vi "Main_14a.vi"() -> ()   [LabVIEW 2023]
uses:
  ENUM_Type.ctl
panel:
  out "End":T1[][](array[typedef])
  out "Start":T1[][](array[typedef])
  out "Answer":i32
  in  "Puzzle":string="O.OO.#...#.O#...#...O..O.#O..O.##.....###O.O##O.O....OO.....##..##.#..O#.........O#..#..O...#O.....O\n.....###.O....#.#O.....##..O##O.......##......O..#..##.#.O#...O...O.O....#.###O.OO#.#O.#.#..O..OOO..\nOO......#.#..##O........O.###..#.#........O#..O....O#.#.##.OO.....O#.........###O......#..#.O..#....\n..#O...O....#.#.#O#....#.O#....OO.OO.O#...O##.O........O.#O.OO.O.....O.#.O.#....O.....O..OO.OO...O.#\n..#O...#.....O#O...###O......O#.##O..O#.O.O.#..#O#.O....O..O#...OO...O..#.O.......O.##OO.#...#...##.\n.#......O.OO#....O#O#OO.O..O......OOO..O....O....#OO....O...#.O.O.O..O...OOOO...#......O..#O..#O....\n..O.#.O.#..OO...........#..#......#.#...#...O...#...#...O##..O..#..O.#...O..#.O...#....#..OO..O..#.#\n.##..O..##O......#...##....#..#..O....#..##.#.O#....O#..#...O.O....O.O.........OO.#.OO......O.......\n..##O.O...O.O..O##OO..#.O..O.#...O..#..#.O...O....##...#O...O......#.....O##O#..O.#..#..O...#...#.O.\nO..##...##...#.#.OO#...OO#O..O...O.#O..#.O......O##......#O..O..OOOOOO..O.##.O...#O.....O##......OO.\n.........O..O#.....#...#......OO###OO.O.O#...#.O....O..##..O#.....O.#.##O.#......#.O.....OO#.#..##O.\nOO#O...#...OO.O####.OO.#.#.......O......O#..O#..#...#O....#.....OO#O......#O#...O#.OO......O....O#..\n.O.........#.#O#....#OO..#.........OO....O...#.O.O.O.OOO.O..O.....O.#....OOOO....OO.......#.#.O.##..\n....#.....#.O.#O...O#OO#...##.#.#..O.O.O....#O.#.#.O...#O#O.O#O...O..#OO..O###.OO..#.....OOO.#......\n#OOO..OO.O.O..O..O....#....O..O.#...O...O...##.O##..O...OOOOO#.........OOO##..#...OO#O#O.....O...##.\n.......O#..#OO.O.O..OO.O#..O.......##....OO#.O..O..O#...#..#...O.##.....#..........#.....#.O...#...O\n......O.#.O...O.......O#..O..OOO#...#........###.O..#....O.O#.OO.O..#.O#O.O.O.......O.##.OO......O.#\nO....O..........#....##.###..#...O#.O..O.##.O....O..O..O..##.O.O#OO...O.#.O##..#.#.......#.O..O..O.O\n..O#..O.#.##..O#..O#..O..O..O....OO...O##..#...O.OO..#.#.#.###O.O...#O.##..#.....#..#O.O.O...#O.O#..\n..O.##........OO.....OO.O..#.....OO.O..#...#..OOO..#....#....#.OO.#.#........OO...O.#O....##O..OOOO#\n.........#.#.OO.#O...#...O#........O..#.#........O......O#.OO..#..#....O##OO.......O..O.O.O.........\n#..O..#..OO.O.O....O..O.O.#.O.O#O...O.OO..#......OO.#..O....#.....#OOO#.OO#.OO........###....O.....O\n..O..O.O.O.....O..#.O..##.O..##..O###........O.O..#...O....OOO#.OO.#O...O..##....#.#O...#..O...O...#\nO#...O..O.#.#......O..O.#OO.....O..#.......O.##O........#O.OO..#..O.##..O.#...O...#O.....#.#..OO##..\nO.OO..O....O.#..O##O.#.O.O#O..##...O..##...#.O#.....O##.#O..O.O.....O....##..O.###......#........O..\n.....##.#.......O.OO....#..##............##..O..#.......O..O..#.O...O#..O.O.##..O..OO.O.....O...O...\n##.O.#....O..OO..OOO.OO.##..OO.OO.#...O#.....#...##...O#....OO..O.O...O...O.#....OO...#..#O#.##..#..\n........OOO....O...#.O...O..#......O....#O#.#O...O#.O........O.O...OO#....O..#.#.#O.O...OO....O.#O..\nOO...O...O..#.OO..O#.OO###..O.......#..O..O.####O....O.O.O#O.#..O..##OO..O..#....#..O#O....#..O...O.\n..O....#.O.O....O...#.........#..O#.#..OO....#...##.OO..OO.O...OOO..O..O#.###.......O#...#....OO...#\n.O...OO.O.O...#.......#.O.O.....O...OOOO.#O.O..O..OOO.OO...............#O...##O..OOO##....#O.O#.##..\nO....O...O.#...........#..#.#OO###O.O...#.O#..O.....O...O....O...#...O.OOO.OO#..OO...#..OOOO...#..#.\n....O...OO.#.O...O..#....O.O.#O..O....O..O..##O.#O....O..O.....O.......OO.......#OO#.##.O.#.O..#.##O\n#OO#.#....###O#..OO..#..O.......O.O...OO#.#O.....O.O##.O...#.##O#...O#......#..#..O#O.O.....OO.O#.O.\n...O#....O...O......#..O#O..OO.O#.OO.#.......#...O..O.....O.#O..O..O.....#OO#.O..#....#O.#O..#......\n..O.....O.......#O....O#...##.....#..O.#....#.#.#O#.#....O....#..O.O......OO....O.#OO#OO.....O......\n.#..O..#..O##...#O.#.##O#.#.#O....O#..###.OO..##..#..........O#O.#..#....O...##.......O.O.O##O#..#O.\n.#.....O..O.#..#..O....O...#.....#O.O.....OO.#..#......##........O.#.#......#...OO#....O#O.....#..O#\n#.....O.....O...O..##O.OO#OO......O#..O......O...O...#.....OO..#...O..#.....##.#.O...#..#O......OO.O\n.#..#.#.#...O#.......#.O....O..#.#.#.....O...................#.O...OOO#.....O.O.....O..O.#.....#.O.O\nO....O.....O.....O#O...O.O.O#O.#O..OO#OO..#OO.OO##.....##O#.O.O..#.....O..OO.##.#.......#...O..OO.O.\n.O#..O..#....##......O....#.#.#......#........##...#....#.......#.....O......##.#.....O.O....OO#.O..\n....OO.OO#...O..#O#O.#.O.#..OO...OOO...#O.#..#..#.#O...#O.#.O..##..O.##..O#.#.....#..O...#.O...O#.O#\n....O#....O.O#OOO...#.#.........O.O....#..O...#...#.....O.O.O.O....#.OO.##O.....#.#.#.#O..O#.O.#.OOO\nO#OO..O.#.......###..OO..O........O.##O.#O##..O...O.#OO.....#...O......O.OO...O..OO....O..O..#.#...O\n.#.O.O.O.#......O......##O...OO.....O....O#.....O#....#.......#O..#...##..O..#O.O.O..O....O.........\n...#.........OO..O.O#..O.#....#...OO##...O..OO.......#.#OO..#...#..##.#...OO#...#O.#...O.....O...#..\n#.....#O......O....O#.....#.#O.OO..........O.O...#....#.###O.O..O...#...#..#....O..O..O#.O.........#\nO.O.O...O...#.....#.#....O.O.O.....OO....#..OOO......O.O.......O#O...#.#O##O.####.........O#O.......\nO.O...........O#...OO..#O.O.O......O.......##.O...O..##...O.#OO...#OO...#...#O#.##O.#......O.##....O\nO..#...........O..O......OOO....#....OO.O...#O..O.O#......#...........#O...#O..O....#.#.#..#...#O...\n..O.....#...#...O.#.O..##.........O#..##.....#O.........................##...#.#..#.OO#O...#OOO#O.##\nOO..O.O.....O#.O....O##...O.O#.OO.#..O.....O...##.O#..O......OO..#..O.....##.....OO#OO...#O......O.O\n.OO...#....#O..#.....OO..O.O.......O#...O#..O#..#.O....#.O.#.O...O.#.O.#...#..OO.......O#....OO..O..\nO.OO..#.OOO.#.O#...#.#..O..O#.#.#.#.....#.O#..O....O..OO...O..#..#....OO#O.#......O#..##...O...O.#O.\n....#....#...OO#...O.O#OO.#.#OOO..O...OO.O..#.O#..#..O.O..#.#........OO#O.#.#.#.....OO......##.#.O..\n.#.O.OOO#OOO...##O#.#...#...##O.#...O.......###O#.##..O#..#.##...O..O.O.........O..#..O##......#.##.\nO...#..#....#O..##..O.O##..O.O###O.......O...#.O#.O#..O...#.#.O..#.....#.....O..O..OOO.OOO..O..OOO..\n...O#.O....O.O.#.O..#.O..####...OO......#OO....O#....O..O...O...OO..OO.OOO#....#..#.O.O..#..#.....O.\nO.O##O.O.O.#.O.#........#O......#O.##...##OO.......O#..#..#.O....OO........#.#O..#O.........OO.O#..O\n.......#.....O...O.O.#O##.O.OO#.....O.O#O....O.#.##.#.......##.O.O.###O...O.O#O##...#...#...O..#....\n.O#...#O...#....O##.O..........O.O.#..O.O..OOOOO.......OO.O#...O...O...#O###OOO.#OOO..............O#\nO.#.#.......OO..OO.#.O#.....#.O#O...#......O....O...O.O.....OO.#O.......#..O...O.....##OO#.....OO#.#\n...O#...#.....#..#O.#..O..O.#O#O.#...OO#O.O....O.#...#O#O....#......O..#O...#....O..O.O........#..#.\n.O.......#..O#...O....................#.##O......#.#......####..OO#...OO.##..#........#.OO..#OOO.###\n......O...O..O##.......O...O##O.O....#..#.##...#OO..##..........#..............##O.......O...#O###O.\n.........#..OO.#.......OO...O....#O.#.......O..##...###..O...#OO.O.O...#...#OO....##O.....#O.O..#...\n..#....O..O......#.#....OO#....#...O.#.OO.O#.....O#.#......O.#O.........O....O....#..O.........O....\n.OO.......#.....O.O..O#....O.#.....O..O#O...O#.....OOO....##..O.O..O#.OO...#....#...O..#..##..#..#.O\nO..#..OO##.#..OOO..#...#.OOO..O..##..O..##O.......O.O..O...#.O...#..###.#.#.#...#O..O......#.O#....#\n...O..#O..O..OO.#....#...##...O...#.......OOOO#...O.###.O.......#O.O#.##.##O..#...O...O.O..#....OO..\nOO.........OO...O.O............O....O.O...O.O.O.......O.OOO.O#....#O.O..#.....O#...#...#....#......O\n#.OO#........OO..#OO.....O.#...#..#O.O...O.....#..O.......O...O..O...O.O.O....##...O....O.OO.....#.O\n..O....#..O....O#.....#..#O......O......#...#O.......O.O...##O.#...O#..O#.#O###...#.OOO.#O...O#....O\n.#.#..OO.#..O###....O.#......O..OO...O.O..O.#.O....O.#..O.....O#....O....#.......O.O...O......OOO.#.\n...OO#.OO#O....O....O.O.#.O.#O..#.O#...###...#......#...OO##.#.#..O#...#....#.#.#.OO....O...OOOO...O\n..O.#..O...O...O#O......##.....O...O..O....#....O..#OO.#.O......#O.OOO.O.O..#........##...#O.#O...O.\n..O.OO.....O...#..O..#...O...O..#O..O#..##.....#....#.#O.#.......#O##....O.OOOOOOOO#.O...O.O#..#O##.\nO.OO.####..OO...OO.O........OO#.O.O...#....#..OO......O.O...O..#.##....O....O......#O........#O.O#..\n.#O.#...#.#...OO#.O.#O.....O##.O.OO.O..#..#O.....O...#.O.O#.....###.....#O.O.......O.#O.O#..#.O..#..\n.O......O........O...#O....##.....#O..OO.O..#.....O.#..O...#O#.#..##.#O..........O.O.O..#....#..#..#\n.OOO..O...#O.O#..#....O......O.O...O#O.....#..OO......OO.#O..O..O###......O.#.#.#.O....#...O........\n.##.....#OO#.##.....#....O..O.....OO..OO##...O...O#.##.OO#....#.......#...O.O.#.O........OO...OO....\n......OO#.....OO#OO......#.O....##..O.O#...O....#..O.O.#O.#...#.O..#.O.O#O....O.O..O.O.O.#OO.##.OO.#\n.O..OO##....O###......####.OO...O#..#..##.##.O..#..##OOO...#..#O##.#..#........#...#....O.......#.OO\n..O..O.O..#....#.#O.#.#OOO....O.##.....OO....#..O...#...#O.........O....O..#..........#.O..O.OO.O##O\nOO.......#...O#.#.......O...O.OO#.O.O.....O.....#...##..#....#.......O#.#O..O.O.......##...OO..#O...\n#O#....#.#.O..#...OO...##.#.#.O#O#...#........O..OO..#..O#..O..O.O.#O...#.....#O.#O.O#..OOO#.O.O..#.\n.#O...OO.##.#.....O...O#O................O.O..O#...#..O.#OO..O....OO...O.#...O#.#.O...O#....OO#.#...\nO#...###.OO.O...O.O#O#..O.O...O.#.....O......O...#...O.O....#...O...O#.#...##....O...........#O...#.\n.....#OO.#.OO...##.O....#OO#.....O..##...OO#.......O...##..#....#..#..##.#O.O##..O.#.O.#.O#OO.O.#.#O\nO##.#..O.OO..O.O.OOO.O...O..O.O..O.O.O..#.........#.....OO.#.......O#....#.......#O.#.O..#...O#..OOO\n.#....O.O..O##...#.OO#.O#..#OO..O.#...O....##.#O.O#O#...#.........O.#..#....OO..O.#........##O.##O..\n.....#....OO#...#.OO.O.O....O..#O.#.O#.O##.O..#.#O.#..O.#.O..O#.#.O.O.O#O....OO#...O......OO#..OO#O.\nO..O.#O..OOO..O...O...#.......#O.OO....O..#...O.....O.#.OO....#.O.OO...O#...OOO###.O..#.....O..O#.#.\n.OO......O#O.......OOO.......O..O...........O..##.....OO..##...O.O.O...O.O.O.....O..OO..O#....#.O..#\nO....#....#O.####.O...#....O....#O..#O...O.O....O.O#..O.........O#.......O....O..O...#.##..O.OO.OO..\n.O###O...#OO.OO........O.O#.O.O....O.O...##.O#..###..........#..O#.O..O.OO.O..#O#OO..O#.O.##.O.OOO##\n#.#O#..O.#...O#..#.......O#..#...#...#O..#.O.....O...O.......#O.#...#OO.O....OO..O...#.#....#O......\n..O.#O.O.O#..#.O...#.....#..O..##..O......O.OO.O.###.....#.O..O...OO#.OO.....#...OO#O..#..#O#...O..O"
  in  "Example":string="O....#....\nO.OO#....#\n.....##...\nOO.#O....O\n.O.....O#.\nO.#..O.#.#\n..O..#O..O\n.......O..\n#....###..\n#OO..#...."
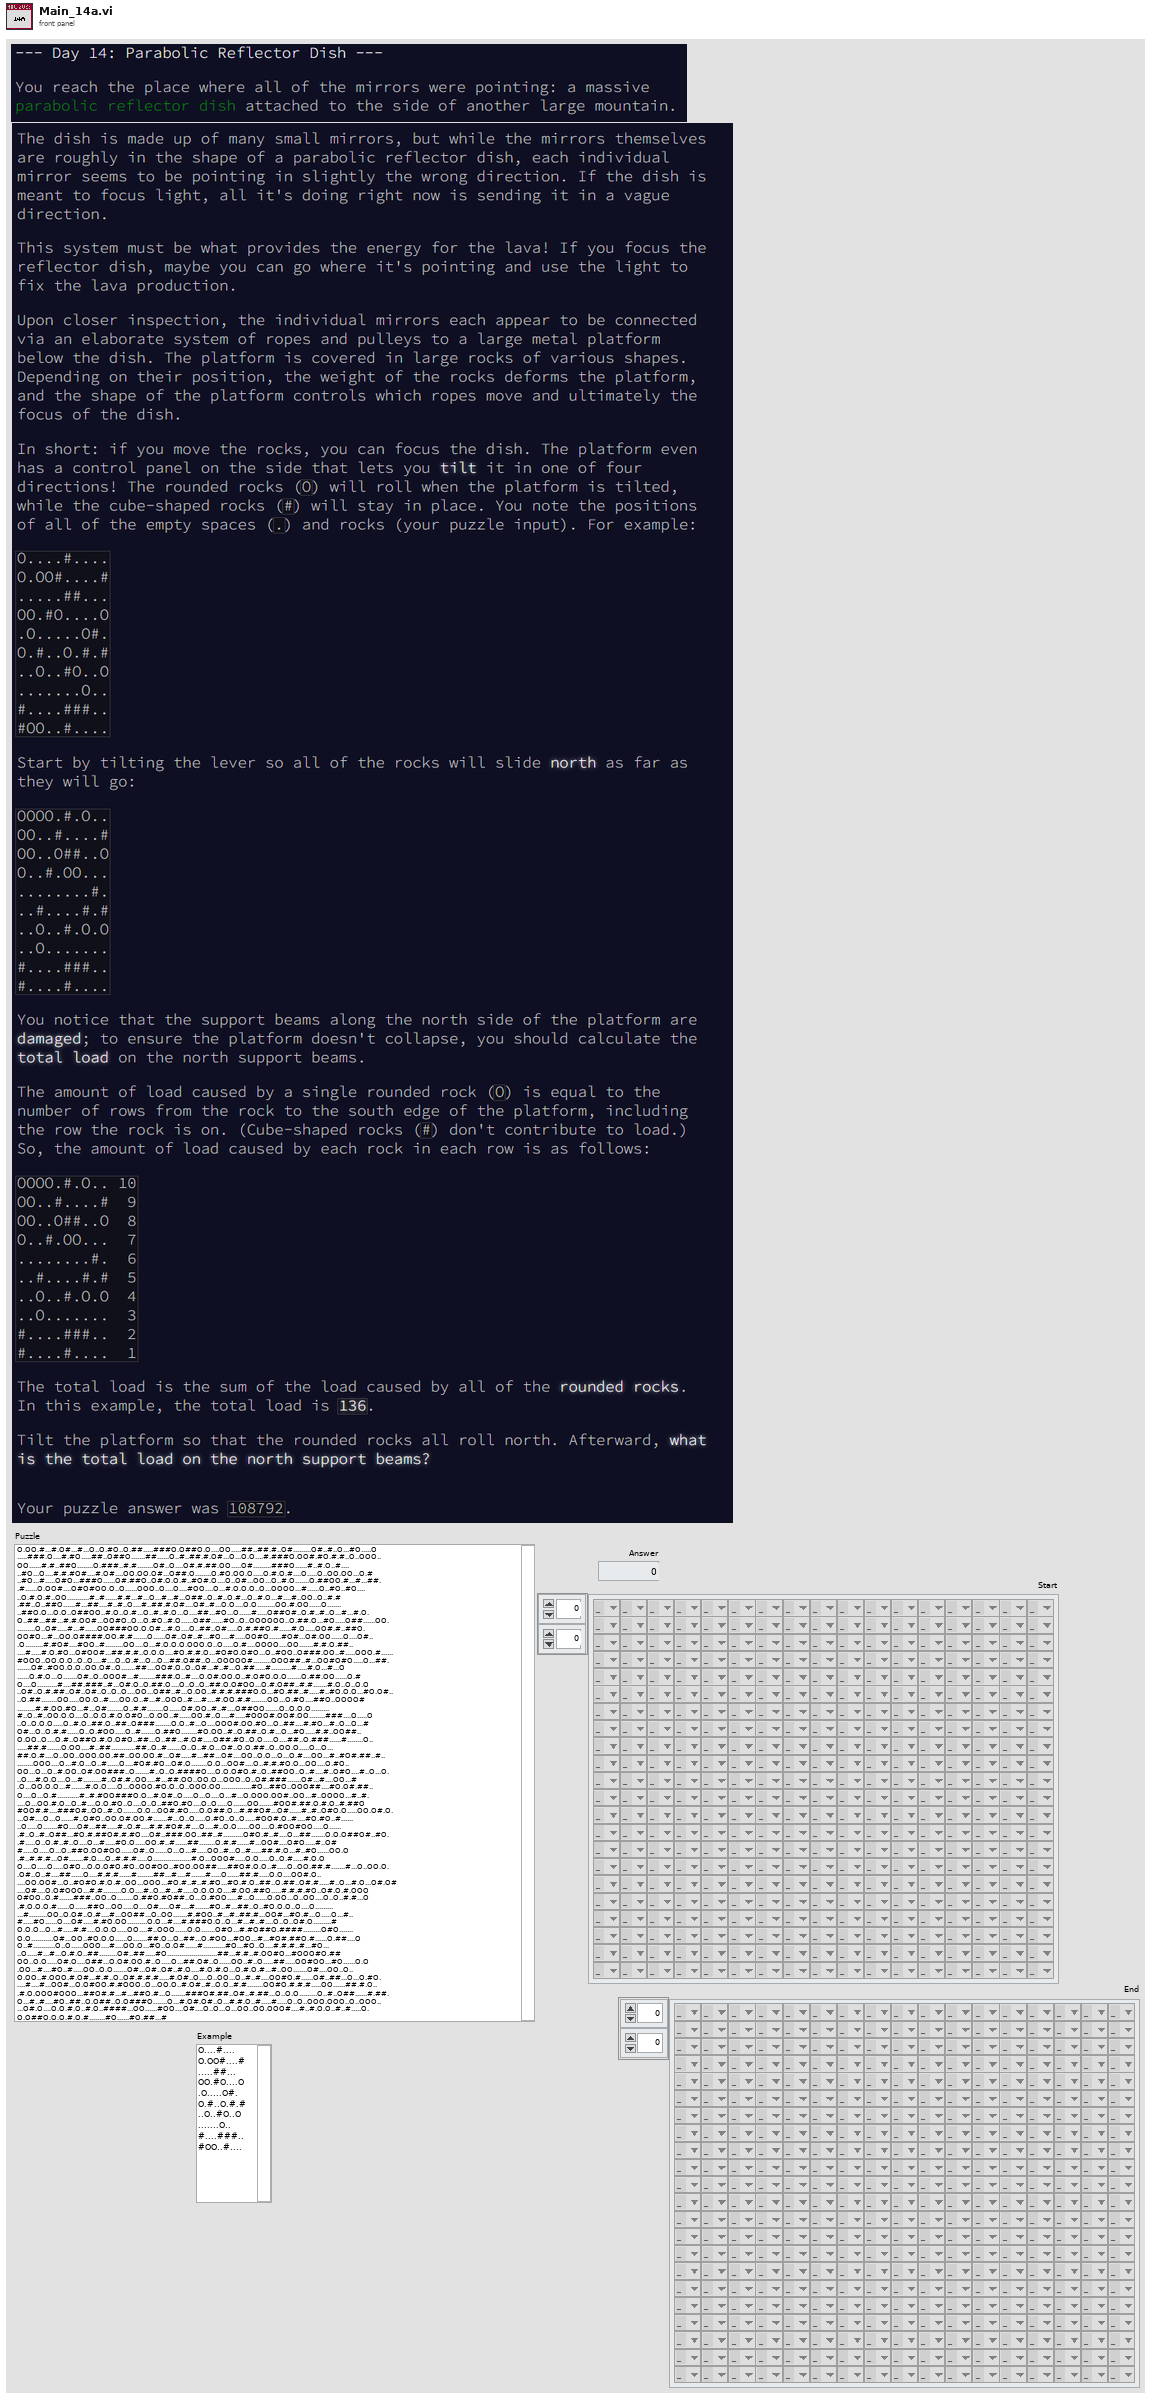
[diagram p1: front panel]
types:
  T1 = typedef "ENUM_Type.ctl" = enum16{"_", "O", "#"}
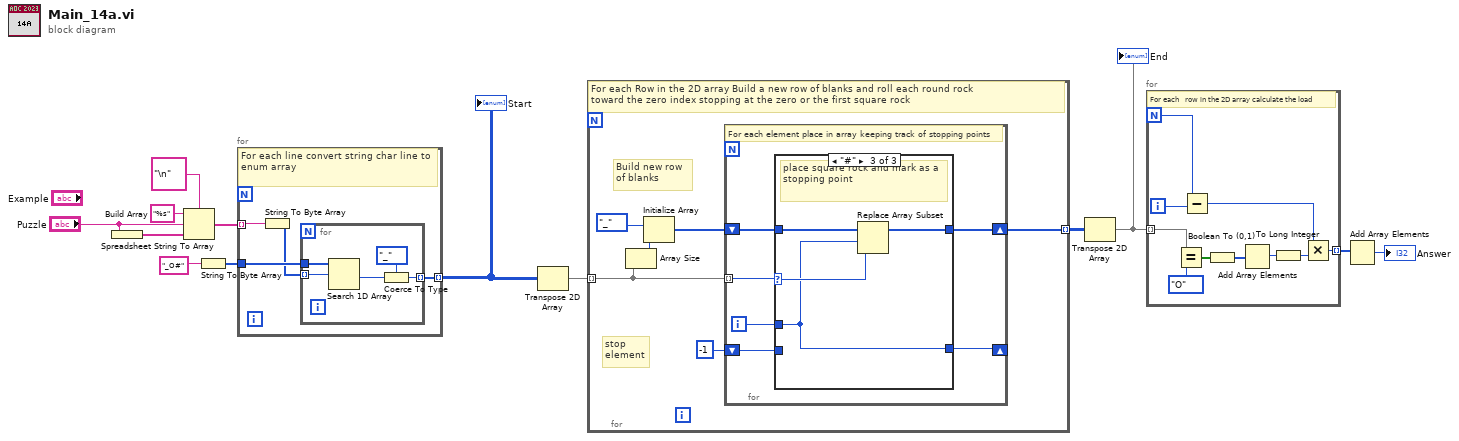
[diagram p0: block diagram]
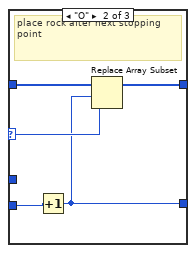
[diagram p3: hidden frame]
diagram:
  n1 = Build Array("Puzzle") -> (w13:string[])
  n2 = Spreadsheet String To Array(delimiter (Tab)="\n", format string="%s", spreadsheet string="Puzzle", array type (2D Dbl)=w13) -> (array=w10:string[])
  n3 = String To Byte Array(string="_O#") -> (unsigned byte array=w8:u8[])
  n4 = for {
    tunnel: w10 -> [w17] mode=indexing
    tunnel: w8 -> [w16]
    tunnel: [w14] -> w7 mode=indexing
    # "For each line convert string char line to enum array"
    n5 = String To Byte Array(string=w17) -> (unsigned byte array=w15:u8[])
    n6 = for {
      tunnel: w16 -> [w22]
      tunnel: w15 -> [w21] mode=indexing
      tunnel: [w18] -> w14 mode=indexing
      n7 = Search 1D Array(1D array=w22, element=w21) -> (index of element=w20:i32)  [unwired: 1 in]
      n8 = Coerce To Type(0:w20, 1:ENUM_Type."_" ("Enum")) -> (2:w18:T1)
    }
  }
  "Start" <- w7
  n9 = Transpose 2D Array(2D array=w7) -> (transposed array=w6:T1[][])
  n10 = for {
    tunnel: w6 -> [w25] mode=indexing
    tunnel: [w23] -> w5 mode=indexing
    # "stop\nelement"
    # "Build new row\nof blanks"
    # "For each Row in the 2D array Build a new row of blanks and roll each round rock\ntoward the zero index stopping at the zero or the first square rock"
    n11 = Array Size(array=w25) -> (size(s)=w27:i32)
    n12 = Initialize Array(ENUM_Type."_" ("Enum"), w27) -> (w26:T1[])
    n13 = for {
      shift-right: [w30] -> w23
      shift-left: w26 -> [w32]
      shift-right: [w31] -> _
      shift-left: -1 -> [w33]
      tunnel: w25 -> [w34] mode=indexing
      i -> [w29]
      # "For each element place in array keeping track of stopping points"
      n14 = case shown="\"#\"" w34 {
        selector: w34 -> [_ w38 w43]
        tunnel: w33 -> [w35 w41 _]
        tunnel: w32 -> [w36 w40 w45]
        tunnel: [w35 w37 w42] -> w31
        tunnel: [w36 w39 w44] -> w30
        tunnel: w29 -> [_ _ w42]
        frame "_" {
          # "Do nothing"
        }
        frame "O" {
          # "place rock after next stopping point"
          n15 = Increment(x=w41) -> (x+1=w37:i32)
          n16 = Replace Array Subset(array=w40, new element=w38, index=w37) -> (w39:T1[])
        }
        frame "#" {
          # "place square rock and mark as a stopping point"
          n17 = Replace Array Subset(array=w45, new element=w43, index=w42) -> (w44:T1[])
        }
      }
    }
  }
  n18 = Transpose 2D Array(2D array=w5) -> (transposed array=w4:T1[][])
  "End" <- w4
  n19 = for {
    N -> [w55]
    tunnel: w4 -> [w53] mode=indexing
    tunnel: [w47] -> w3 mode=indexing
    i -> [w54]
    # "For each   row in the 2D array calculate the load"
    n20 = Equal?(x=w53, y=ENUM_Type."O" ("Enum")) -> (x = y?=w51:bool[])
    n21 = Subtract(x=w55, y=w54) -> (x-y=w48:i32)
    n22 = Boolean To (0,1)(Boolean=w51) -> (0, 1=w50:i16[])
    n23 = Add Array Elements(numeric array=w50) -> (sum=w49:i16)
    n24 = To Long Integer(number=w49) -> (32bit integer=w46:i32)
    n25 = Multiply(x=w48, y=w46) -> (x*y=w47:i32)
  }
  n26 = Add Array Elements(numeric array=w3) -> (sum=→"Answer":i32)
